vi "Cal11-RunMeasurement.vi"(0 "String in":refnum<vi>, 1 "reference in":refnum<vi>, 2 "Results file output":path, 3 "Din":dbl[](array[numeric]), 4 "CIn":dbl[](array[numeric]), 6 "EIn":dbl[](array[numeric]), 7 "BIn":dbl[](array[numeric]), 8 "data mode":enum16{"Take new data point", "Refit Curve"}(ring), 9 "Ain":dbl[](array[numeric]), 11 "-ve Ref Values":bool) -> (10 "Aout":dbl[](array[numeric]), 12 "BOut":dbl[](array[numeric]), 13 "Status Out":T1, 14 "COut":dbl[](array[numeric]), 15 "Dout":dbl[](array[numeric]), 16 "EOut":dbl[](array[numeric]), 17 "String":string, 18 "Sample of input signals":dbl[][](graph))   [LabVIEW 2022 SP3]
uses:
  Anemometry Sub Vis/Gen Trav/Multi_Run_Status.ctl
  Anemometry Sub Vis/Controls/Setup.ctl
  Anemometry Sub Vis/Controls/Post_Process.ctl
  Anemometry Sub Vis/Controls/Save_Data.ctl
  <vilib>/Analysis/baseanly.llb/Mean (DBL).vi
  Anemometry Sub Vis/Globals/Calib_global.vi
  Anemometry Sub Vis/Globals/Meas_global.vi
  Anemometry Sub Vis/Acquisition/PWA/PWAtasksGLOBAL.vi
  <vilib>/Analysis/NI_AALBase.lvlib
  <vilib>/Analysis/NI_AALPro.lvlib
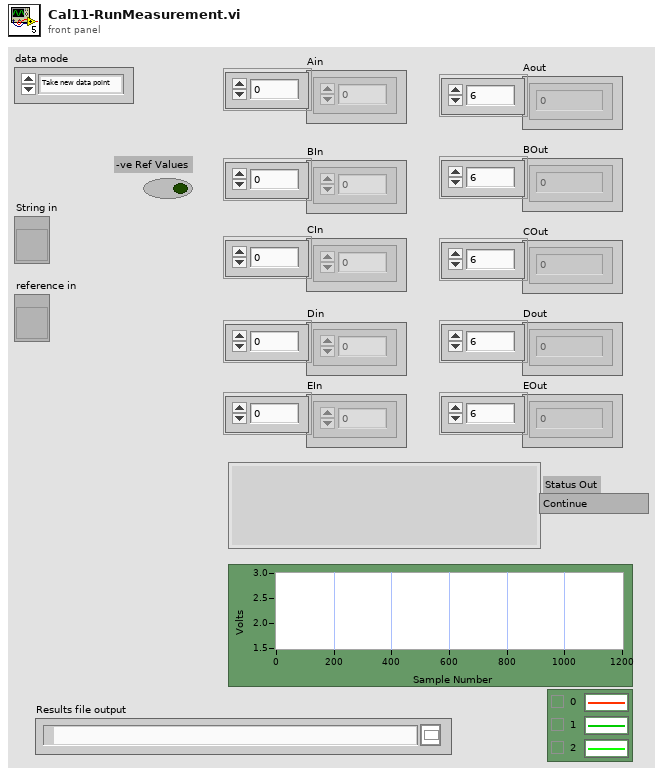
[diagram p1: front panel]
types:
  T1 = typedef "Multi_Run_Status.ctl" = enum16{"Continue", "Continue with Error", "Jump to Next Point", "Jump to Next Row", "Jump To Fall Back", "Terminate Run"}
  T2 = typedef "Ref_Inst_type.ctl" = enum16{"Propellor anemometer", "Pressure Transducer", "Raw voltage", "Pitot-static tube", "Generic Linear", "Generic Polynomial", "Thermocouple", "LDA", "Enter Value", "ADAM Channel"}
  T3 = cluster{"2nd Ref type":T2, "2nd inst present":bool}
  T4 = typedef "Cal_Inst_type.ctl" = enum16{"Propeller anemometer", "Pressure Transducer", "Hot wire", "Cross wire velocity", "Cross wire angle", "Generic Linear", "Generic Polynomial", "Poly Fit Special", "Fast FID", "Thermocouple", "Cold wire", "Pulsed Wire"}
  T5 = typedef "Save_Data.ctl" = enum16{"Save No Data", "Save Data"}
  T6 = typedef "Post_Process.ctl" = enum16{"Take New Data", "Post Process Raw Data File"}
  T7 = typedef "Setup.ctl" = enum16{"Run Program", "Show Setup", "Save Current Setup", "Setup Front Panel"}
  T8 = typedef "Time_Trace_Cluster.ctl" = cluster{"Weighting":dbl[], "Voltage":dbl[], "Eng Values":dbl[]}
  T9 = typedef "Analysis_info_cluster.ctl" = cluster{"Colour":u32, "Inst type":T10, "Inst name":string, "Symbol":string, "Code name":string, "Extra Info":string, "Inst Array":T11, "Extra Titles":string[], "Extra Values":string[], "U":dbl, "u^2":dbl, "u^3":dbl, "u^4":dbl, "Skew_u":dbl, "Kurt_u":dbl, "Sd Error in Mean":dbl, "% u'/U":dbl, "X":dbl, "Y":dbl, "Z":dbl, "Timescale integral Estimate":dbl, "Sd Error in Variance":dbl, "Calib File":path, "Calib Constants":dbl[], "Output Position":bool, "Stats":enum16{"None", "Basic", "Full"}, "Av Sampling Rate":dbl, "Av No of Samples":dbl, "Total Meas Time (s)":dbl, "ADAM Ch Name":string, "Max value":dbl, "Min value":dbl, "Req Sample Rate Hz":dbl, "Sync Delay Time (s)":dbl, "Ch No":i16, "Device":string, "Use Latest Calib":bool, "Port":string, "Metadata Ch Names":string[], "Metadata Ch Values":string[], "Label":string, "chState":T12}
  T10 = typedef "Inst_type.ctl" = enum16{"Raw voltage", "Raw with zero offsetting", "Propeller anemometer", "Pressure Transducer", "Pitot-static tube", "Hot wire", "Cross wire 1", "Cross wire 2", "Generic Linear", "Generic Polynomial", "Generic BackPoly", "Fast FID", "Thermocouple", "Cold wire", "Pulsed Wire", "LDA Vel", "LDA Tran time", "LDA Arr time", "Microphone"}
  T11 = typedef "Instrument_Array.ctl" = enum16{"PWA", "LDA", "Analogue"}
  T12 = typedef "channelState.ctl" = enum32{"No Selection", "Solo", "Mute"}
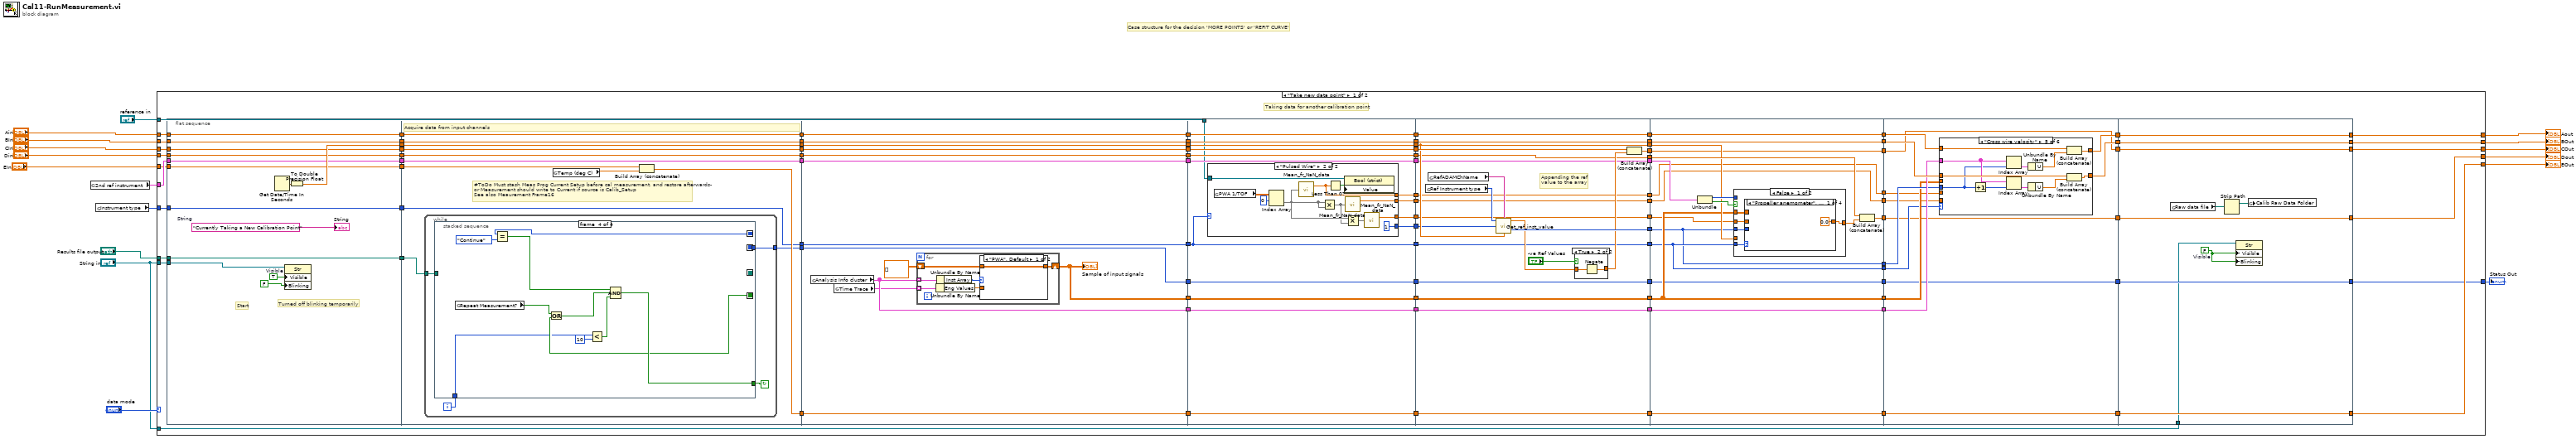
[diagram p0: block diagram]
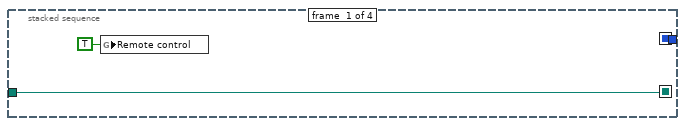
[diagram p2: hidden frame]
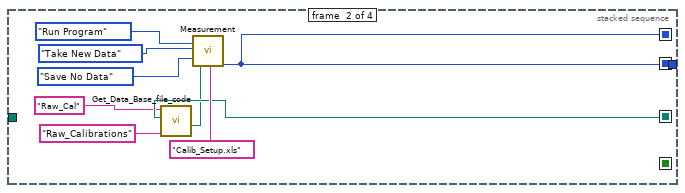
[diagram p3: hidden frame]
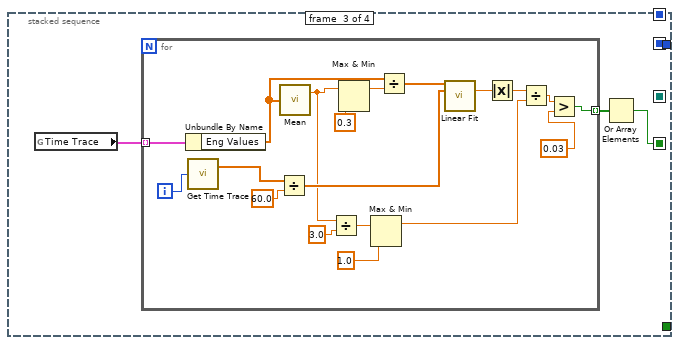
[diagram p4: hidden frame]
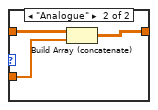
[diagram p5: hidden frame]
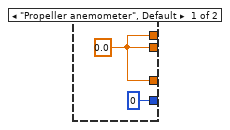
[diagram p6: hidden frame]
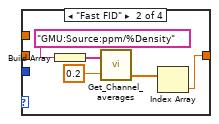
[diagram p8: hidden frame]
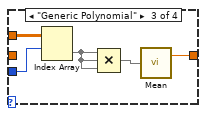
[diagram p9: hidden frame]
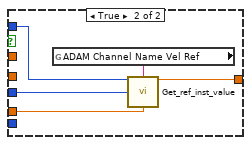
[diagram p11: hidden frame]
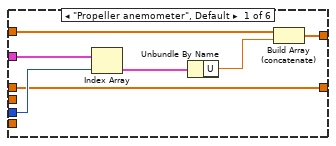
[diagram p12: hidden frame]
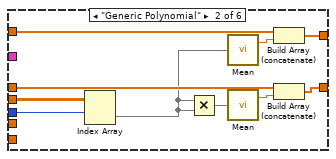
[diagram p13: hidden frame]
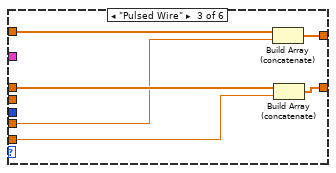
[diagram p14: hidden frame]
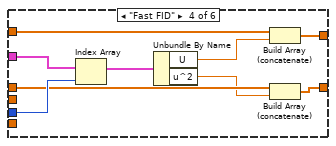
[diagram p15: hidden frame]
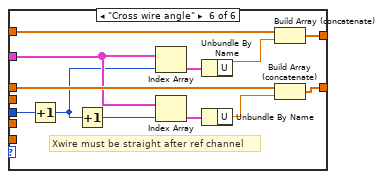
[diagram p16: hidden frame]
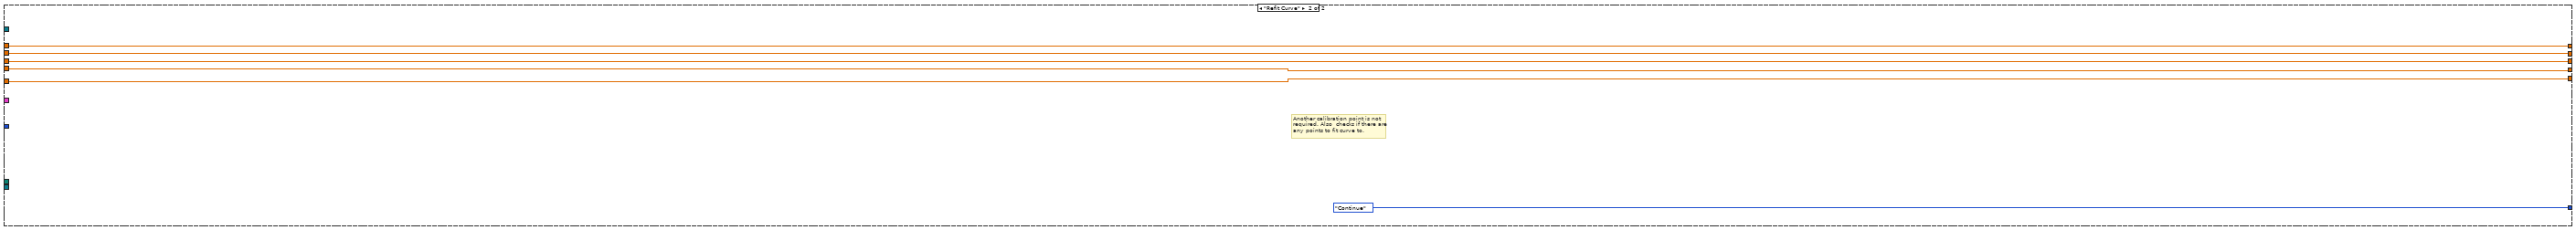
[diagram p17: hidden frame]
diagram:
  # "Case structure for the decision 'MORE POINTS' or 'REFIT CURVE'"
  n1 = global read "Calib_global.vi" "2nd ref instrument"() -> (w11:T3)
  n2 = global read "Calib_global.vi" "Instrument type"() -> (w16:T4)
  n3 = case shown="\"Take new data point\"" "data mode" {
    tunnel: [w108 w388] -> w6
    tunnel: [w109 w384] -> w5
    tunnel: "Ain" -> [w110 w388]
    tunnel: "CIn" -> [w111 w384]
    tunnel: [w107 w387] -> w7
    tunnel: "BIn" -> [w106 w387]
    tunnel: "Din" -> [w105 w386]
    tunnel: [w103 w386] -> w10
    tunnel: w11 -> [w104 _]
    tunnel: [w101 w385] -> w12
    tunnel: "EIn" -> [w102 w385]
    tunnel: "Results file output" -> [w100 _]
    tunnel: [w99 Multi_Run_Status."Continue" ("Status Out")] -> w13
    tunnel: w16 -> [w98 _]
    tunnel: "String in" -> [w20 _]
    tunnel: "reference in" -> [w19 _]
    tunnel: "String in" -> [w18 _]
    frame "Take new data point" {
      # "Taking data for another calibration point"
      # "Start"
      n4 = flat-sequence {
        tunnel: w110 -> [w122]
        tunnel: [w122] -> w97
        tunnel: w111 -> [w121]
        tunnel: [w121] -> w96
        tunnel: w106 -> [w120]
        tunnel: [w120] -> w95
        tunnel: w105 -> [w119]
        tunnel: [w119] -> w94
        tunnel: w104 -> [w118]
        tunnel: [w118] -> w93
        tunnel: w102 -> [w117]
        tunnel: [w117] -> w92
        tunnel: w100 -> [w116]
        tunnel: [w116] -> w91
        tunnel: w98 -> [w115]
        tunnel: [w115] -> w90
        tunnel: [w125] -> w89
        tunnel: w20 -> [w113]
        tunnel: w97 -> [w132]
        tunnel: [w132] -> w88
        tunnel: w96 -> [w131]
        tunnel: [w131] -> w87
        tunnel: w95 -> [w130]
        tunnel: [w130] -> w86
        tunnel: w94 -> [w129]
        tunnel: [w129] -> w85
        tunnel: w93 -> [w128]
        tunnel: [w128] -> w84
        tunnel: w92 -> [w137]
        tunnel: [w136] -> w83
        tunnel: w91 -> [w134]
        tunnel: [w135] -> w82
        tunnel: w90 -> [w127]
        tunnel: [w127] -> w81
        tunnel: w89 -> [w126]
        tunnel: [w126] -> w80
        tunnel: w88 -> [w195]
        tunnel: [w195] -> w79
        tunnel: w87 -> [w194]
        tunnel: [w194] -> w78
        tunnel: w86 -> [w193]
        tunnel: [w193] -> w77
        tunnel: w85 -> [w192]
        tunnel: [w192] -> w76
        tunnel: w84 -> [w191]
        tunnel: [w191] -> w75
        tunnel: w83 -> [w190]
        tunnel: [w190] -> w74
        tunnel: w82 -> [w189]
        tunnel: [w189] -> w73
        tunnel: w81 -> [w188]
        tunnel: [w188] -> w72
        tunnel: w80 -> [w187]
        tunnel: [w187] -> w71
        tunnel: [w198] -> w70
        tunnel: [w186] -> w69
        tunnel: w79 -> [w220]
        tunnel: [w220] -> w68
        tunnel: w78 -> [w219]
        tunnel: [w219] -> w67
        tunnel: w77 -> [w218]
        tunnel: [w218] -> w66
        tunnel: w76 -> [w217]
        tunnel: [w217] -> w65
        tunnel: w75 -> [w216]
        tunnel: [w216] -> w64
        tunnel: w74 -> [w215]
        tunnel: [w215] -> w63
        tunnel: w73 -> [w214]
        tunnel: [w214] -> w62
        tunnel: w72 -> [w223]
        tunnel: [w223] -> w61
        tunnel: w71 -> [w213]
        tunnel: [w213] -> w60
        tunnel: w70 -> [w212]
        tunnel: [w212] -> w59
        tunnel: w69 -> [w211]
        tunnel: [w211] -> w58
        tunnel: [w224] -> w57
        tunnel: [w222] -> w56
        tunnel: [w221] -> w55
        tunnel: [w210] -> w54
        tunnel: w19 -> [w209]
        tunnel: w68 -> [w249]
        tunnel: [w249] -> w53
        tunnel: [w259] -> w52
        tunnel: w67 -> [w258]
        tunnel: w66 -> [w248]
        tunnel: [w248] -> w51
        tunnel: w65 -> [w247]
        tunnel: [w247] -> w50
        tunnel: w64 -> [w246]
        tunnel: [w246] -> w49
        tunnel: w63 -> [w245]
        tunnel: [w245] -> w48
        tunnel: w62 -> [w244]
        tunnel: [w244] -> w47
        tunnel: w61 -> [w243]
        tunnel: [w243] -> w46
        tunnel: [w256] -> w45
        tunnel: w60 -> [w257]
        tunnel: [w257] -> w44
        tunnel: w59 -> [w242]
        tunnel: [w242] -> w43
        tunnel: w58 -> [w241]
        tunnel: [w241] -> w42
        tunnel: w57 -> [w252]
        tunnel: w56 -> [w240]
        tunnel: [w240] -> w41
        tunnel: w55 -> [w239]
        tunnel: [w239] -> w40
        tunnel: w54 -> [w238]
        tunnel: [w238] -> w39
        tunnel: w53 -> [w271]
        tunnel: [w271] -> w38
        tunnel: w52 -> [w270]
        tunnel: [w270] -> w37
        tunnel: w51 -> [w269]
        tunnel: [w269] -> w36
        tunnel: w50 -> [w278]
        tunnel: [w277] -> w35
        tunnel: w49 -> [w276]
        tunnel: w48 -> [w268]
        tunnel: [w268] -> w34
        tunnel: w47 -> [w264]
        tunnel: [w264] -> w33
        tunnel: w46 -> [w273]
        tunnel: [w273] -> w32
        tunnel: w45 -> [w263]
        tunnel: w44 -> [w275]
        tunnel: w43 -> [w267]
        tunnel: [w267] -> w31
        tunnel: [w263] -> w30
        tunnel: w42 -> [w274]
        tunnel: [w274] -> w29
        tunnel: w41 -> [w266]
        tunnel: [w266] -> w28
        tunnel: w40 -> [w265]
        tunnel: [w265] -> w27
        tunnel: w39 -> [w272]
        tunnel: w38 -> [w317]
        tunnel: w37 -> [w307]
        tunnel: [w307] -> w26
        tunnel: [w316] -> w25
        tunnel: [w315] -> w24
        tunnel: w36 -> [w314]
        tunnel: w35 -> [w306]
        tunnel: [w306] -> w23
        tunnel: w34 -> [w305]
        tunnel: [w305] -> w22
        tunnel: w33 -> [w304]
        tunnel: [w304] -> w21
        tunnel: w32 -> [w310]
        tunnel: w31 -> [w313]
        tunnel: w30 -> [w312]
        tunnel: w29 -> [w311]
        tunnel: w28 -> [w309]
        tunnel: w27 -> [w308]
        tunnel: [w380] -> w109
        tunnel: w26 -> [w380]
        tunnel: [w379] -> w108
        tunnel: w25 -> [w379]
        tunnel: [w378] -> w107
        tunnel: w24 -> [w378]
        tunnel: [w377] -> w103
        tunnel: w23 -> [w377]
        tunnel: [w376] -> w101
        tunnel: w22 -> [w376]
        tunnel: [w375] -> w99
        tunnel: w21 -> [w375]
        tunnel: w18 -> [w373]
        frame #0 {
          w123 = TRUE  # Visible
          w114 = "Currently Taking a New Calibration Point"  # String
          # "Turned off blinking temporarily"
          n5 = Get Date/Time In Seconds() -> (seconds since 1Jan1904=w124:timestamp)
          n6 = property on="Property Node" class="Str"(reference=w113, "Visible"=w123, "Blinking"=FALSE) -> ()  [unwired: 1 in, 2 out]
          n7 = To Double Precision Float(number=w124) -> (double precision float=w125:dbl)
          "String" <- w114
        }
        frame #1 {
          # "#ToDo Must stash Meas Prog Current Setup before cal measurement, and restore afterwards- or Measurement should write to Current if source is Calib_Setup\nSee also Meaurement Frame16"
          # "Acquire data from input channels"
          n8 = while {
            tunnel: [w141] -> w135
            tunnel: w134 -> [w140]
            i -> [w138]
            stop <- w139 continue-if-true
            n9 = stacked-sequence {
              seq-local: [w142 _ _ _] -> [_ w149 _ _]
              seq-local: [_ w145 _ _] -> [_ _ _ w181]
              seq-local: [_ w145 _ _] -> [_ _ _ w182]
              seq-local: [_ _ w153 _] -> [_ _ _ w179]
              tunnel: w140 -> [w142 _ _ _]
              tunnel: [_ _ _ w181] -> w141
              tunnel: [_ _ _ w183] -> w139
              tunnel: w138 -> [_ _ _ w177]
              frame #0 {
                n10 = global write "Meas_global.vi" "Remote control"(TRUE ("Remote control")) -> ()
              }
              frame #1 {
                n11 = call "Get_Data_Base_file_code.vi"("Data Type"="Raw_Calibrations", "Results Filename"=w149, "Short_Name"="Raw_Cal" ("Data Type")) -> ("Raw Data File Name"=w146:path)  [unwired: 1 in, 3 out]
                n12 = call "Measurement.vi"("setup"=Setup."Run Program", "Post Process"=Post_Process."Take New Data", "File"=Save_Data."Save No Data", "Raw data file"=w146, "Setup filename"="Calib_Setup.xls") -> ("Status Out"=w145:T1)  [unwired: 1 in, 13 out]
              }
              frame #2 {
                n13 = global read "Meas_global.vi" "Time Trace"() -> (w155:T8[])
                n14 = for {
                  tunnel: w155 -> [w170] mode=indexing
                  tunnel: [w156] -> w154 mode=indexing
                  i -> [w169]
                  n15 = Unbundle By Name(w170) -> ("Eng Values"=w174:dbl[])
                  n16 = call "Get Time Trace.vi"("Channel Index"=w169) -> ("Time (s)"=w167:dbl[])  [unwired: 1 out]
                  n17 = Divide(x=w167, y=60.0) -> (x/y=w166:dbl[])
                  n18 = call-poly <vilib>:"Mean.vi"("X"=w174) -> ("mean"=w162:dbl)  [unwired: 1 out]
                  n19 = Divide(x=w162, y=3.0) -> (x/y=w164:dbl)
                  n20 = Max & Min(x=w162, y=0.3) -> (max(x,y)=w173:dbl)  [unwired: 1 out]
                  n21 = Max & Min(x=w164, y=1.0) -> (max(x,y)=w159:dbl)  [unwired: 1 out]
                  n22 = Divide(x=w174, y=w173) -> (x/y=w171:dbl[])
                  n23 = call <vilib>:"Linear Fit.vi"("Y"=w171, "X"=w166) -> ("slope"=w161:dbl)  [unwired: 9 in, 4 out]
                  n24 = Absolute Value(x=w161) -> (abs(x)=w160:dbl)
                  n25 = Divide(x=w160, y=w159) -> (x/y=w158:dbl)
                  n26 = Greater?(x=w158, y=0.03) -> (0:w156:bool)
                }
                n27 = Or Array Elements(Boolean array=w154) -> (logical OR=w153:bool)
              }
              frame #3 {
                n28 = global read "Meas_global.vi" "Repeat Measurement?"() -> (w180:bool)
                n29 = Equal?(x=w182, y=Multi_Run_Status."Continue" ("Status Out")) -> (x = y?=w184:bool)
                n30 = Or(x=w180, y=w179) -> (x .or. y?=w178:bool)
                n31 = Less?(x=w177, y=10) -> (x < y?=w175:bool)
                n32 = Compound Arithmetic op=AND(w184, w178, w175) -> (w183:bool)
              }
            }
          }
          n33 = global read "Calib_global.vi" "Temp (deg C)"() -> (w133:dbl)
          n34 = Build Array (concatenate)(w137, w133) -> (w136:dbl[])
        }
        frame #2 {
          n35 = global read "Meas_global.vi" "Analysis Info cluster"() -> (w198:T9[])
          n36 = global read "Meas_global.vi" "Time Trace"() -> (w196:T8[])
          n37 = for {
            tunnel: w198 -> [w204] mode=indexing
            shift-right: [w201] -> w186
            shift-left: dbl[][] [] -> [w202]
            tunnel: w196 -> [w200] mode=indexing
            n38 = Unbundle By Name(w200) -> ("Eng Values"=w199:dbl[])
            n39 = Unbundle By Name(w204) -> ("Inst Array"=w203:T11)
            n40 = case shown="\"PWA\", Default" w203 {
              tunnel: w202 -> [w205 w208]
              tunnel: w199 -> [_ w207]
              tunnel: [w205 w206] -> w201
              frame "PWA", Default {
              }
              frame "Analogue" {
                n41 = Build Array (concatenate)(w208, w207) -> (w206:dbl[][])
              }
            }
          }
          "Sample of input signals" <- w186
        }
        frame #3 {
          n42 = case shown="\"Pulsed Wire\"" w223 {
            tunnel: [0 ("Index in") 1 ("Index in")] -> w224
            tunnel: [w225 w229] -> w222
            tunnel: [w225 w233] -> w221
            tunnel: [w225 w232] -> w210
            tunnel: w209 -> [_ w227]
            frame "Propeller anemometer", Default {
              w225 = 0.0 ("mean")
            }
            frame "Pulsed Wire" {
              n43 = global read "PWAtasksGLOBAL.vi" "PWA 1/TOF"() -> (w236:dbl[][])
              n44 = Index Array(array=w236, index (row)=0) -> (element=w234:dbl[])  [unwired: 1 in]
              n45 = call "Mean_fr_NaN_data.vi"("Data"=w234) -> ("Mean value"=w229:dbl)  [unwired: 1 out]
              n46 = Multiply(x=w234, y=w234) -> (x*y=w231:dbl[])
              n47 = Less Than 0?(x=w229) -> (x < 0?=w228:bool)
              n48 = property class="Bool (strict)"(reference=w227, "Value"=w228) -> ()  [unwired: 1 in, 2 out]
              n49 = call "Mean_fr_NaN_data.vi"("Data"=w231) -> ("Mean value"=w233:dbl)  [unwired: 1 out]
              n50 = Multiply(x=w234, y=w231) -> (x*y=w230:dbl[])
              n51 = call "Mean_fr_NaN_data.vi"("Data"=w230) -> ("Mean value"=w232:dbl)  [unwired: 1 out]
            }
          }
        }
        frame #4 {
          # "Appending the ref\nvalue to the array"
          n52 = global read "Calib_global.vi" "Ref Instrument type"() -> (w255:T2)
          n53 = global read "Calib_global.vi" "RefADAMChName"() -> (w250:string)
          n54 = call "Get_ref_inst_value.vi"("Ref Instrument type"=w255, "ADAM Channel Name"=w250, "Index in"=w252, "Start time"=w257) -> ("Ref Value"=w254:dbl, "Index out"=w256:i32)  [unwired: 3 in, 7 out]
          n55 = case shown="True" "-ve Ref Values" {
            tunnel: w254 -> [w260 w262]
            tunnel: [w260 w261] -> w253
            frame False {
            }
            frame True {
              n56 = Negate(x=w262) -> (-x=w261:dbl)
            }
          }
          n57 = Build Array (concatenate)(w258, w253) -> (w259:dbl[])
        }
        frame #5 {
          n58 = Unbundle(w276) -> ("2nd Ref type"=w280:T2, "2nd inst present"=w279:bool)
          n59 = case shown="False" w279 {
            tunnel: w263 -> [w286 w300]
            tunnel: [w284 w301] -> w281
            tunnel: w280 -> [_ w302]
            tunnel: w275 -> [_ w303]
            tunnel: w274 -> [w285 _]
            tunnel: w273 -> [w283 _]
            tunnel: w272 -> [w282 _]
            frame False {
              n60 = case shown="\"Propeller anemometer\", Default" w283 {
                tunnel: w286 -> [_ _ w297 _]
                tunnel: w285 -> [_ _ w296 _]
                tunnel: [0.0 ("mean") w288 w294 w298] -> w284
                tunnel: w282 -> [_ _ _ w298]
                frame "Propeller anemometer", Default {
                }
                frame "Fast FID" {
                  n61 = Build Array("GMU:Source:ppm/%Density") -> (w291:string[])
                  n62 = call "Get_Channel_averages.vi"("Desired Ch Names"=w291, "Averaging time (mins)"=0.2) -> ("number"=w289:dbl[])  [unwired: 1 in, 2 out]
                  n63 = Index Array(array=w289) -> (element=w288:dbl)  [unwired: 1 in]
                }
                frame "Generic Polynomial" {
                  n64 = Index Array(array=w296, index (row)=w297) -> (element=w293:dbl[])  [unwired: 1 in]
                  n65 = Compound Arithmetic op=MULTIPLY(w293, w293, w293) -> (w295:dbl[])
                  n66 = call-poly <vilib>:"Mean.vi"("X"=w295) -> ("mean"=w294:dbl)  [unwired: 1 out]
                }
                frame "Pulsed Wire" {
                }
              }
            }
            frame True {
              n67 = global read "Calib_global.vi" "ADAM Channel Name Vel Ref"() -> (w299:string)
              n68 = call "Get_ref_inst_value.vi"("Ref Instrument type"=w302, "ADAM Channel Name"=w299, "Index in"=w300, "Start time"=w303) -> ("Ref Value"=w301:dbl)  [unwired: 4 in, 7 out]
            }
          }
          n69 = Build Array (concatenate)(w278, w281) -> (w277:dbl[])
        }
        frame #6 {
          n70 = case shown="\"Cross wire velocity\"" w310 {
            tunnel: w317 -> [w322 w332 w339 w347 w359 w371]
            tunnel: [w323 w333 w340 w348 w360 w372] -> w316
            tunnel: w314 -> [w321 w331 w338 w343 w358 w370]
            tunnel: [w321 w330 w337 w341 w357 w369] -> w315
            tunnel: w313 -> [w319 _ _ w345 w353 w365]
            tunnel: w312 -> [w324 w334 _ w349 w350 w363]
            tunnel: w311 -> [_ w329 _ _ _ _]
            tunnel: w309 -> [_ _ w336 _ _ _]
            tunnel: w308 -> [_ _ w335 _ _ _]
            frame "Propeller anemometer", Default {
              n71 = Index Array(array=w319, index=w324) -> (element=w320:T9)
              n72 = Unbundle By Name(w320) -> ("U"=w318:dbl)
              n73 = Build Array (concatenate)(w322, w318) -> (w323:dbl[])
            }
            frame "Generic Polynomial" {
              n74 = Index Array(array=w329, index (row)=w334) -> (element=w326:dbl[])  [unwired: 1 in]
              n75 = Multiply(x=w326, y=w326) -> (x*y=w325:dbl[])
              n76 = call-poly <vilib>:"Mean.vi"("X"=w326) -> ("mean"=w328:dbl)  [unwired: 1 out]
              n77 = call-poly <vilib>:"Mean.vi"("X"=w325) -> ("mean"=w327:dbl)  [unwired: 1 out]
              n78 = Build Array (concatenate)(w332, w328) -> (w333:dbl[])
              n79 = Build Array (concatenate)(w331, w327) -> (w330:dbl[])
            }
            frame "Pulsed Wire" {
              n80 = Build Array (concatenate)(w339, w336) -> (w340:dbl[])
              n81 = Build Array (concatenate)(w338, w335) -> (w337:dbl[])
            }
            frame "Fast FID" {
              n82 = Index Array(array=w345, index=w349) -> (element=w346:T9)
              n83 = Unbundle By Name(w346) -> ("U"=w344:dbl, "u^2"=w342:dbl)
              n84 = Build Array (concatenate)(w347, w344) -> (w348:dbl[])
              n85 = Build Array (concatenate)(w343, w342) -> (w341:dbl[])
            }
            frame "Cross wire velocity" {
              n86 = Increment(x=w350) -> (x+1=w351:i32)
              n87 = Index Array(array=w353, index=w350) -> (element=w356:T9)
              n88 = Index Array(array=w353, index=w351) -> (element=w355:T9)
              n89 = Unbundle By Name(w356) -> ("U"=w352:dbl)
              n90 = Unbundle By Name(w355) -> ("U"=w354:dbl)
              n91 = Build Array (concatenate)(w359, w352) -> (w360:dbl[])
              n92 = Build Array (concatenate)(w358, w354) -> (w357:dbl[])
            }
            frame "Cross wire angle" {
              # "Xwire must be straight after ref channel"
              n93 = Increment(x=w363) -> (x+1=w361:i32)
              n94 = Increment(x=w361) -> (x+1=w362:i32)
              n95 = Index Array(array=w365, index=w361) -> (element=w368:T9)
              n96 = Index Array(array=w365, index=w362) -> (element=w367:T9)
              n97 = Unbundle By Name(w368) -> ("U"=w364:dbl)
              n98 = Unbundle By Name(w367) -> ("U"=w366:dbl)
              n99 = Build Array (concatenate)(w371, w364) -> (w372:dbl[])
              n100 = Build Array (concatenate)(w370, w366) -> (w369:dbl[])
            }
          }
        }
        frame #7 {
          w374 = FALSE  # Visible
          n101 = global read "Meas_global.vi" "Raw data file"() -> (w382:path)
          n102 = Strip Path(path=w382) -> (stripped path=w381:path)  [unwired: 1 out]
          n103 = property on="Property Node" class="Str"(reference=w373, "Visible"=w374, "Blinking"=w374) -> ()  [unwired: 1 in, 2 out]
          n104 = global write "Calib_global.vi" "Calib Raw Data Folder"(w381) -> ()
        }
      }
    }
    frame "Refit Curve" {
      # "Another calibration point is not\nrequired. Also  checks if there are\nany points to fit curve to."
    }
  }
  "Status Out" <- w13
  "EOut" <- w12
  "Dout" <- w10
  "BOut" <- w7
  "Aout" <- w6
  "COut" <- w5
